vi "Convert Tag Bus to Signal.vi"(10 "signal mapping":T2[](array[typedef]), 11 "data table in in":T1) -> (2 "Signal":dbl[](array[numeric]), 3 "data table out":T1)   [LabVIEW 2017, in "J1939 runtime.lvclass"]
uses:
  J1939 runtime.lvclass
  configuration/Signal Mapping.ctl
  <vilib>/NI/Tag Bus/tag/Data Type.ctl
  <vilib>/NI/Tag Bus/table/data table.ctl
  <vilib>/NI/Tag Bus/table/data polymorphs/read one/read Double.vi
  <vilib>/NI/Tag Bus/table/data polymorphs/read one/read Single.vi
  <vilib>/NI/Tag Bus/table/data polymorphs/read one/read I64.vi
  <vilib>/NI/Tag Bus/table/data polymorphs/read one/read I32.vi
  <vilib>/NI/Tag Bus/table/data polymorphs/read one/read I16.vi
  <vilib>/NI/Tag Bus/table/data polymorphs/read one/read I8.vi
  <vilib>/NI/Tag Bus/table/data polymorphs/read one/read U64.vi
  <vilib>/NI/Tag Bus/table/data polymorphs/read one/read U32.vi
  <vilib>/NI/Tag Bus/table/data polymorphs/read one/read U16.vi
  <vilib>/NI/Tag Bus/table/data polymorphs/read one/read U8.vi
  <vilib>/NI/Tag Bus/table/data polymorphs/read one/read Boolean.vi
  <vilib>/NI/Tag Bus/table/data table.lvlib
  <vilib>/NI/Tag Bus/tag/tag descriptor.lvclass
  configuration/J1939 configuration.lvclass
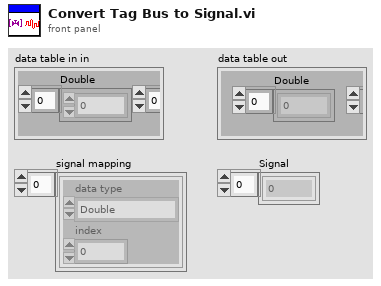
[diagram p1: front panel]
types:
  T1 = typedef "tag bus.lvlib/data table.lvlib/data table.ctl" = cluster{"Double":dbl[], "Single":sgl[], "I64":i64[], "I32":i32[], "I16":i16[], "I8":i8[], "U64":u64[], "U32":u32[], "U16":u16[], "U8":u8[], "Boolean":bool[], "String":string[], "Array of Double":cluster{"DBL Array":dbl[]}[], "Array of Single":cluster{"SGL Array":sgl[]}[], "Array of I64":cluster{"I64 Array":i64[]}[], "Array of I32":cluster{"I32 Array":i32[]}[], "Array of I16":cluster{"I16 Array":i16[]}[], "Array of I8":cluster{"I8 Array":i8[]}[], "Array of U64":cluster{"U64 Array":u64[]}[], "Array of U32":cluster{"U32 Array":u32[]}[], "Array of U16":cluster{"U16 Array":u16[]}[], "Array of U8":cluster{"U8 Array":u8[]}[], "Array of Boolean":cluster{"Boolean Array":bool[]}[], "Array of String":cluster{"String Array":string[]}[]}
  T2 = typedef "J1939 configuration.lvclass/Signal Mapping.ctl" = cluster{"data type":T3, "index":i32}
  T3 = typedef "tag bus.lvlib/tag descriptor.lvclass/Data Type.ctl" = enum16{"Double", "Single", "I64", "I32", "I16", "I8", "U64", "U32", "U16", "U8", "Boolean", "String", "Array of Double", "Array of Single", "Array of I64", "Array of I32", "Array of I16", "Array of I8", "Array of U64", "Array of U32", "Array of U16", "Array of U8", "Array of Boolean", "Array of String"}
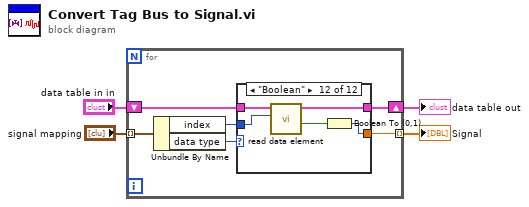
[diagram p0: block diagram]
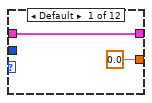
[diagram p2: hidden frame]
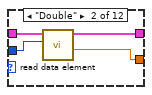
[diagram p3: hidden frame]
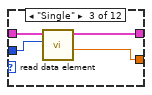
[diagram p4: hidden frame]
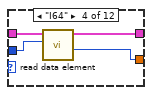
[diagram p5: hidden frame]
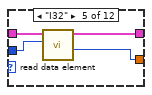
[diagram p6: hidden frame]
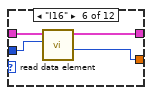
[diagram p7: hidden frame]
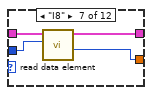
[diagram p8: hidden frame]
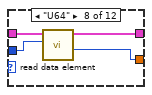
[diagram p9: hidden frame]
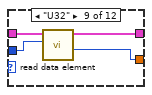
[diagram p10: hidden frame]
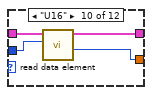
[diagram p11: hidden frame]
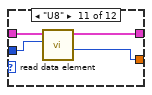
[diagram p12: hidden frame]
diagram:
  n1 = for {
    shift-right: [w8] -> w2
    shift-left: "data table in in" -> [w7]
    tunnel: "signal mapping" -> [w10] mode=indexing
    tunnel: [w6] -> w3 mode=indexing
    n2 = Unbundle By Name(w10) -> ("index"=w5:i32, "data type"=w9:T3)
    n3 = case shown="\"Boolean\"" w9 {
      tunnel: [w12 w15 w19 w23 w27 w31 w35 w39 w43 w47 w51 w56] -> w8
      tunnel: w7 -> [w12 w16 w20 w24 w28 w32 w36 w40 w44 w48 w52 w57]
      tunnel: [0.0 w13 w17 w21 w25 w29 w33 w37 w41 w45 w49 w54] -> w6
      tunnel: w5 -> [_ w14 w18 w22 w26 w30 w34 w38 w42 w46 w50 w55]
      frame Default {
      }
      frame "Double" {
        n4 = call-poly <vilib>:"read data element.vi"("index"=w14, "data table in"=w16) -> ("value"=w13:dbl, "data table out"=w15:T1)  [unwired: 8 in]
      }
      frame "Single" {
        n5 = call-poly <vilib>:"read data element.vi"("index"=w18, "data table in"=w20) -> ("value"=w17:sgl, "data table out"=w19:T1)  [unwired: 8 in]
      }
      frame "I64" {
        n6 = call-poly <vilib>:"read data element.vi"("index"=w22, "data table in"=w24) -> ("value"=w21:i64, "data table out"=w23:T1)  [unwired: 8 in]
      }
      frame "I32" {
        n7 = call-poly <vilib>:"read data element.vi"("index"=w26, "data table in"=w28) -> ("value"=w25:i32, "data table out"=w27:T1)  [unwired: 8 in]
      }
      frame "I16" {
        n8 = call-poly <vilib>:"read data element.vi"("index"=w30, "data table in"=w32) -> ("value"=w29:i16, "data table out"=w31:T1)  [unwired: 8 in]
      }
      frame "I8" {
        n9 = call-poly <vilib>:"read data element.vi"("index"=w34, "data table in"=w36) -> ("value"=w33:i8, "data table out"=w35:T1)  [unwired: 8 in]
      }
      frame "U64" {
        n10 = call-poly <vilib>:"read data element.vi"("index"=w38, "data table in"=w40) -> ("value"=w37:u64, "data table out"=w39:T1)  [unwired: 8 in]
      }
      frame "U32" {
        n11 = call-poly <vilib>:"read data element.vi"("index"=w42, "data table in"=w44) -> ("value"=w41:u32, "data table out"=w43:T1)  [unwired: 8 in]
      }
      frame "U16" {
        n12 = call-poly <vilib>:"read data element.vi"("index"=w46, "data table in"=w48) -> ("value"=w45:u16, "data table out"=w47:T1)  [unwired: 8 in]
      }
      frame "U8" {
        n13 = call-poly <vilib>:"read data element.vi"("index"=w50, "data table in"=w52) -> ("value"=w49:u8, "data table out"=w51:T1)  [unwired: 8 in]
      }
      frame "Boolean" {
        n14 = call-poly <vilib>:"read data element.vi"("index"=w55, "data table in"=w57) -> ("value"=w53:bool, "data table out"=w56:T1)  [unwired: 8 in]
        n15 = Boolean To (0,1)(Boolean=w53) -> (0, 1=w54:i16)
      }
    }
  }
  "Signal" <- w3
  "data table out" <- w2
